vi "PSRDOP.vi"(8 "error in":errorcluster, 10 "String":string, 11 "array":path[](array[path])) -> (0 "error out 8":errorcluster)   [LabVIEW 2025]
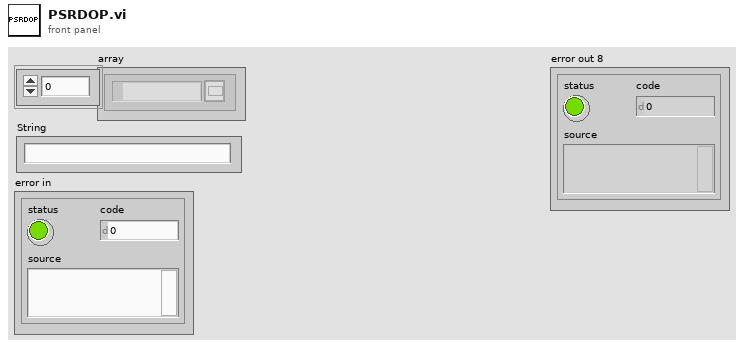
[diagram p1: front panel]
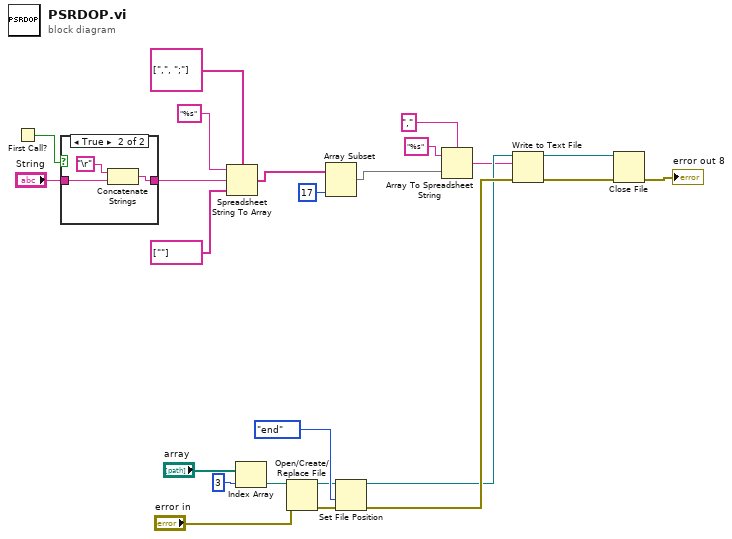
[diagram p0: block diagram]
diagram:
  n1 = First Call?() -> (First Call?: T/F=w8:bool)
  n2 = case shown="True" w8 {
    tunnel: [w25 w27] -> w7
    tunnel: "String" -> [w25 w26]
    frame False {
    }
    frame True {
      n3 = Concatenate Strings("\r", w26) -> (w27:string)
    }
  }
  n4 = Spreadsheet String To Array(delimiter (Tab)=string[] [",", ";"], format string="%s", spreadsheet string=w7, array type (2D Dbl)=string[] [""]) -> (array=w3:string[])
  n5 = Index Array(array="array", index=3 ("index (row)")) -> (element=w14:path)
  n6 = Open/Create/Replace File(file path (use dialog)=w14, error in="error in") -> (refnum out=w15:refnum<file>, error out=w18:errorcluster)  [unwired: 4 in, 1 out]
  n7 = Array Subset(array=w3, length=17) -> (w2:string[])  [unwired: 1 in]
  n8 = Set File Position(refnum=w15, from (0:start)=enum16{"start", "end", "current"}."end", error in=w18) -> (refnum out=w16:refnum<file>, error out=w17:errorcluster)  [unwired: 1 in]
  n9 = Array To Spreadsheet String(delimiter (Tab)=",", array=w2, 3:"%s" ("format string")) -> (spreadsheet string=w11:string)
  n10 = Write to Text File(file (use dialog)=w16, text=w11, error in=w17) -> (refnum out=w20:refnum<file>, error out=w19:errorcluster)  [unwired: 1 in, 1 out]
  n11 = Close File(refnum=w20, error in=w19) -> (error out=→"error out 8":errorcluster)  [unwired: 1 out]
